vi "test-serial.vi"() -> ()   [LabVIEW 2016]
panel:
  out "read buffer":string
  in  "stop":bool
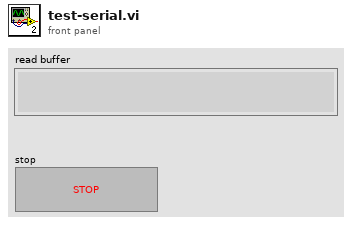
[diagram p1: front panel]
types:
  T1 = cluster{"baud rate (9600)":u32, "data bits (8)":u16, "stop bits (10: 1 bit)":u16, "parity (0:none)":enum16{"None", "Odd", "Even", "Mark", "Space"}, "flow control (0:none)":u16, "timeout (10sec)":u32, "Enable Termination\nChar (T)":bool, "termination char\n(0xA = '\\n' = LF)\n(0xD = '\\r' = CF) ":u8}
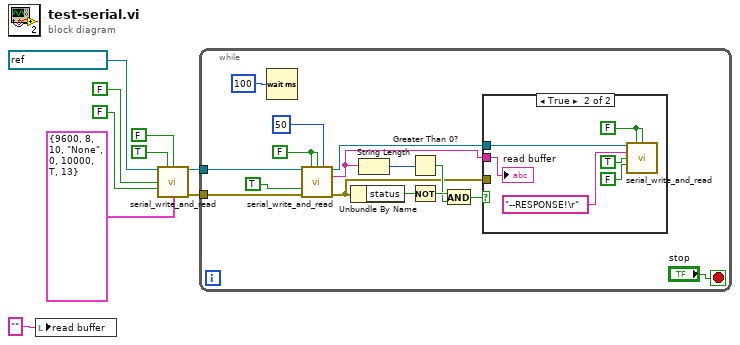
[diagram p0: block diagram]
diagram:
  n1 = local write "read buffer"("" ("read buffer")) -> ()
  n2 = call "serial_write_and_read.vi"("port name in"=refnum<visa-resource-name> "ASRL1::INSTR", "reconnect?"=TRUE, "disconnect?"=FALSE, "do writing?"=FALSE, "expecting response?"=FALSE, "connection parameters"=T1 {"baud rate (9600)"=9600, "data bits (8)"=8, "stop bits (10: 1 bit)"=10, "parity (0:none)"=enum."None", "flow control (0:none)"=0, "timeout (10sec)"=10000, "Enable Termination\nChar (T)"=TRUE, "termination char\n(0xA = '\\n' = LF)\n(0xD = '\\r' = CF) "=13}) -> ("port name out"=w3:refnum<visa-resource-name>, "error out"=w4:errorcluster)  [unwired: 7 in, 1 out]
  n3 = while {
    tunnel: w4 -> [w19]
    tunnel: w3 -> [w23]
    stop <- "stop" stop-if-true
    w18 = FALSE ("disconnect?")
    n4 = Wait (ms)(milliseconds to wait=u32 100) -> ()  [unwired: 1 out]
    n5 = call "serial_write_and_read.vi"("port name in"=w23, "reconnect?"=w18, "disconnect?"=w18, "timeout (ms)"=u32 50, "expecting response?"=TRUE, "error in"=w19) -> ("port name out"=w11:refnum<visa-resource-name>, "read buffer"=w12:string, "error out"=w10:errorcluster)  [unwired: 7 in]
    n6 = Unbundle By Name(w10) -> ("status"=w16:bool)
    n7 = String Length(string=w12) -> (length=w17:i32)
    n8 = Greater Than 0?(x=w17) -> (x > 0?=w13:bool)
    n9 = Not(x=w16) -> (.not. x?=w14:bool)
    n10 = And(x=w14, y=w13) -> (x .and. y?=w15:bool)
    n11 = case shown="True" w15 {
      tunnel: w12 -> [_ w26]
      tunnel: w11 -> [_ w30]
      tunnel: w10 -> [_ _]
      frame False {
      }
      frame True {
        w29 = FALSE ("reconnect?")
        n12 = call "serial_write_and_read.vi"("port name in"=w30, "reconnect?"=w29, "disconnect?"=w29, "write buffer"="--RESPONSE!\r" ("string"), "do writing?"=TRUE, "expecting response?"=FALSE) -> ()  [unwired: 7 in, 3 out]
        "read buffer" <- w26
      }
    }
  }
